vi "Misc.vi"() -> ()   [LabVIEW 2018]
uses:
  <vilib>/Rock Robotics/WPI/DriverStation/WPI_DriverStationRobotMode2.ctl
  <vilib>/Rock Robotics/Network Tables/NT Read Boolean.vi
  SubSystems/Drive Train/Drive Train Global.vi
  <vilib>/Rock Robotics/Network Tables/NT Read String.vi
  Robot Global Data.vi
  SubSystems/HAB Climber/HAB Climber Global.vi
  <vilib>/Rock Robotics/Network Tables/NT Write Boolean.vi
  SubSystems/Lift/Lift Global.vi
  SubSystems/Cargo Intake/Cargo Intake Global.vi
  SubSystems/Hatch Panel Intake/Hatch Panel Intake Global.vi
  <vilib>/Rock Robotics/Network Tables/NT Write Number.vi
  <vilib>/Rock Robotics/Network Tables/NT Write Numeric Array.vi
  Test Mode/Test Mode Global.vi
  <vilib>/Rock Robotics/Network Tables/NT Write Boolean Array.vi
  SubSystems/Controllers/Driver Controller/Driver Controller Global.vi
  SubSystems/Controllers/Manipulator Controlller/Manipulator Controller Global.vi
panel:
  in  "Boolean":bool=TRUE
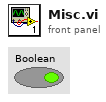
[diagram p1: front panel]
types:
  T1 = typedef "WPI_DriverStationRobotMode2.ctl" = enum16{"Autonomous Disabled", "Autonomous Enabled", "Teleop Disabled", "Teleop Enabled", "Disconnected", "Finish", "Test Disabled", "Test Enabled", "Emergency Stopped"}
  T2 = typedef "WPI_CompressorDevRef.ctl" = cluster{"DevStatus":errorcluster, "Pneumatics Control Module":u8}
  T3 = cluster{"FrontLeft":dbl, "FrontRight":dbl, "BackLeft":dbl, "BackRight":dbl}
  T4 = cluster{"Rollover":dbl, "Yaw":dbl, "Cont Yaw":dbl}
  T5 = cluster{"Drive Test?":bool, "Cargo Test?":bool, "Hatch Test?":bool, "Lift Test?":bool}
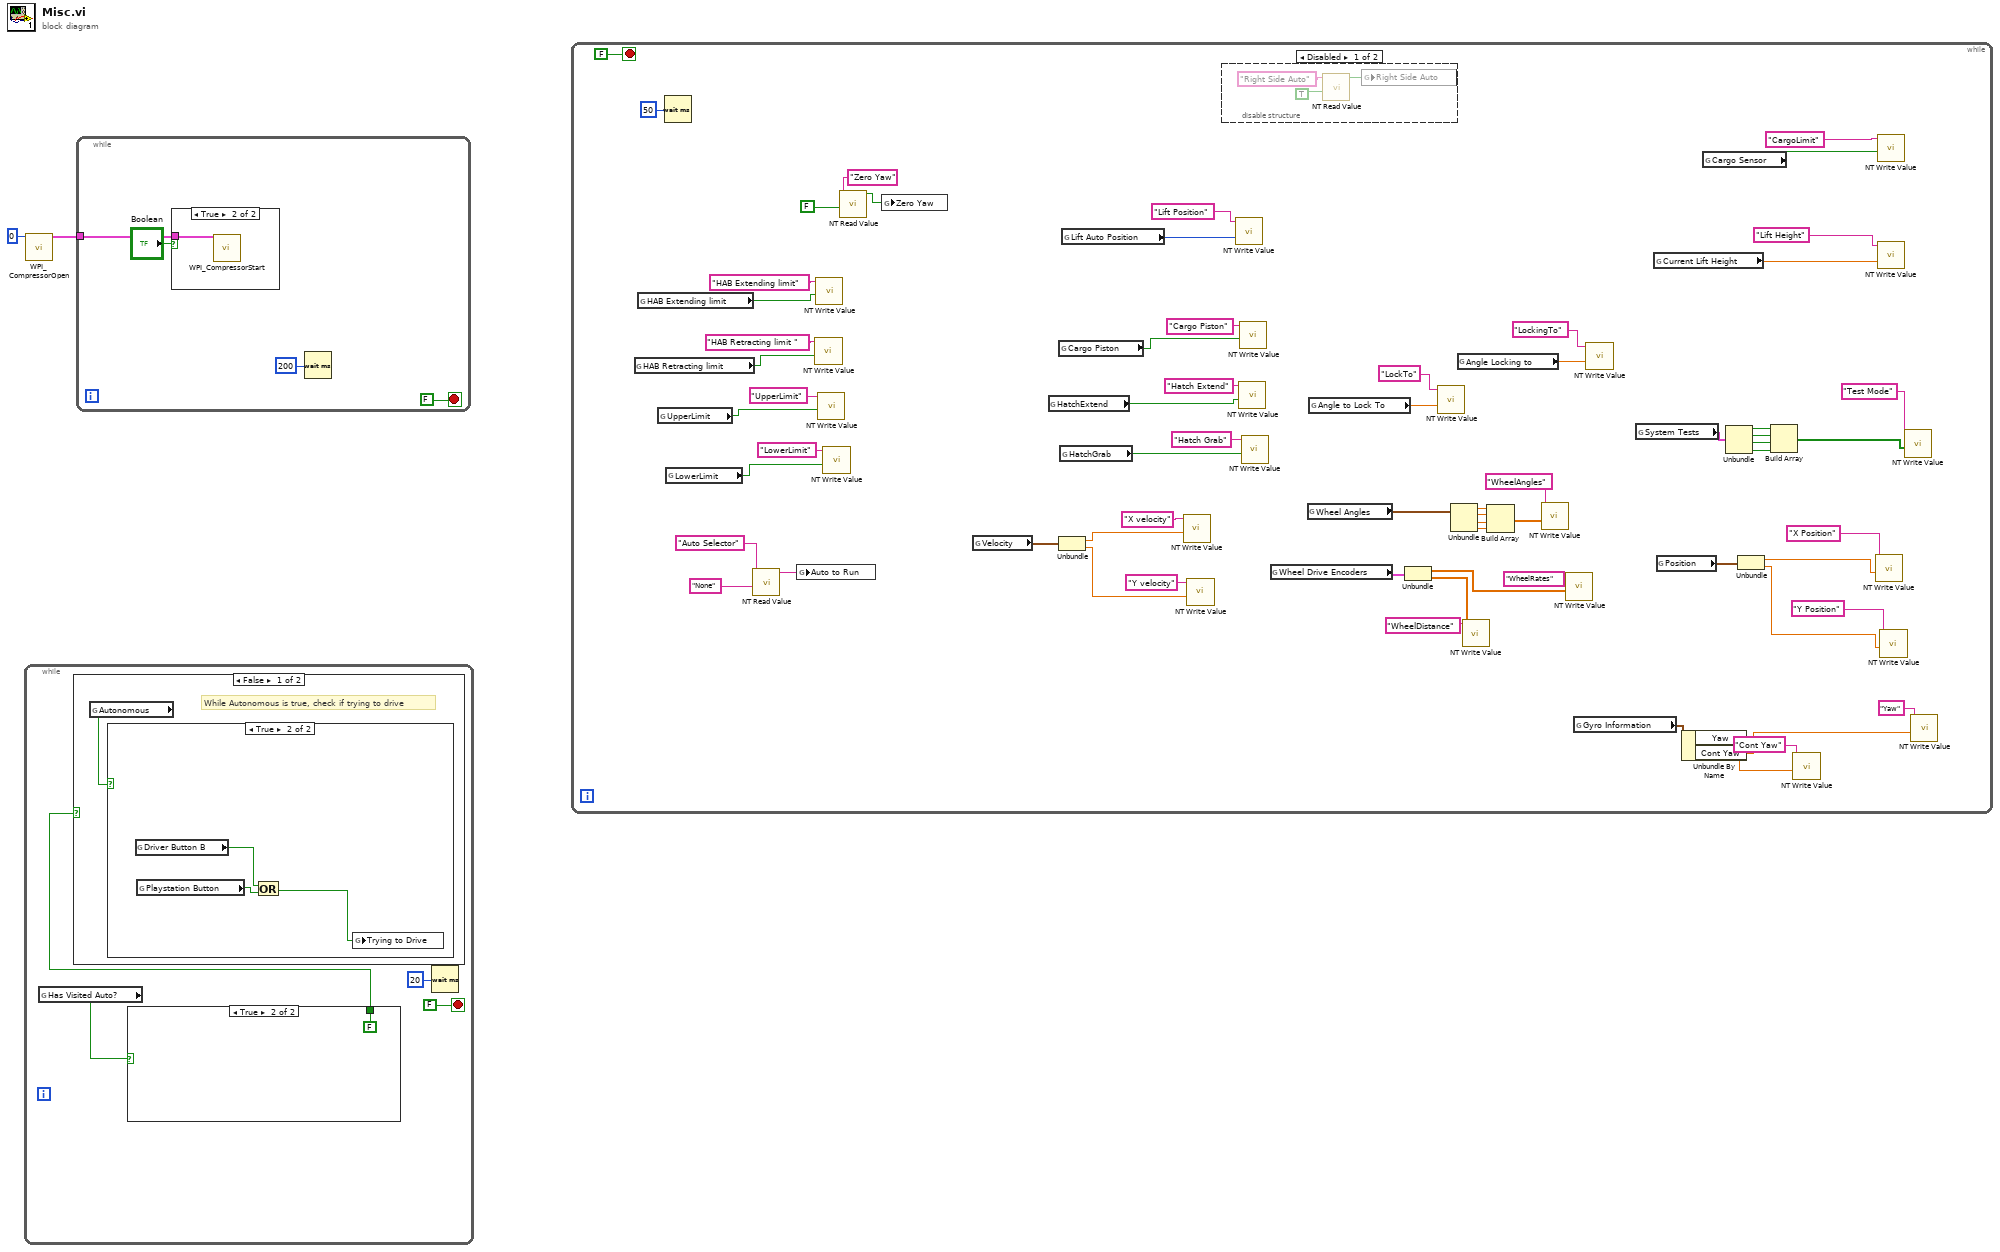
[diagram p0: block diagram]
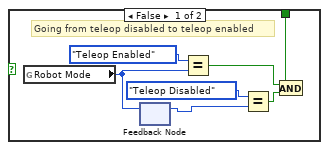
[diagram p2: hidden frame]
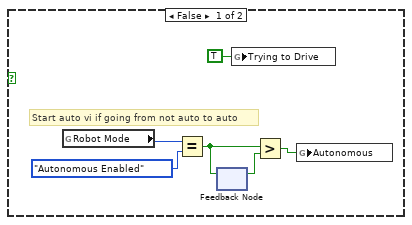
[diagram p3: hidden frame]
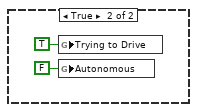
[diagram p4: hidden frame]
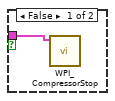
[diagram p6: hidden frame]
diagram:
  n1 = while {
    stop <- FALSE stop-if-true
    n2 = global read "Robot Global Data.vi" "Has Visited Auto?"() -> (w3:bool)
    n3 = case shown="True" w3 {
      tunnel: [w7 FALSE] -> w4
      frame False {
        # "Going from teleop disabled to teleop enabled"
        n4 = global read "Robot Global Data.vi" "Robot Mode"() -> (w13:T1)
        n5 = feedback #1() -> (w10:T1)  [unwired: 1 in]
        n6 = feedback-in #1(w13) -> ()
        n7 = Equal?(x=WPI_DriverStationRobotMode2."Teleop Enabled" ("y"), y=w13) -> (x = y?=w8:bool)
        n8 = Equal?(x=WPI_DriverStationRobotMode2."Teleop Disabled" ("y"), y=w10) -> (x = y?=w9:bool)
        n9 = And(x=w8, y=w9) -> (x .and. y?=w7:bool)
      }
      frame True {
      }
    }
    n10 = case shown="False" w4 {
      frame False {
        # "While Autonomous is true, check if trying to drive"
        n11 = global read "Robot Global Data.vi" "Autonomous"() -> (w15:bool)
        n12 = case shown="True" w15 {
          frame False {
            # "Start auto vi if going from not auto to auto"
            n13 = global read "Robot Global Data.vi" "Robot Mode"() -> (w17:T1)
            n14 = Equal?(x=w17, y=WPI_DriverStationRobotMode2."Autonomous Enabled") -> (x = y?=w18:bool)
            n15 = feedback #2() -> (w19:bool)  [unwired: 1 in]
            n16 = feedback-in #2(w18) -> ()
            n17 = global write "Robot Global Data.vi" "Trying to Drive"(TRUE ("Trying to Drive")) -> ()
            n18 = Greater?(x=w18, y=w19) -> (0:w20:bool)
            n19 = global write "Robot Global Data.vi" "Autonomous"(w20) -> ()
          }
          frame True {
            n20 = global read "Driver Controller Global.vi" "Driver Button B"() -> (w23:bool)
            n21 = global read "Manipulator Controller Global.vi" "Playstation Button"() -> (w22:bool)
            n22 = Compound Arithmetic op=OR(w23, w22) -> (w24:bool)
            n23 = global write "Robot Global Data.vi" "Trying to Drive"(w24) -> ()
          }
        }
      }
      frame True {
        n24 = global write "Robot Global Data.vi" "Trying to Drive"(TRUE ("Trying to Drive")) -> ()
        n25 = global write "Robot Global Data.vi" "Autonomous"(FALSE ("Autonomous")) -> ()
      }
    }
    n26 = Wait (ms)(milliseconds to wait=u32 20) -> ()  [unwired: 1 out]
  }
  n27 = call <vilib>:"WPI_CompressorOpen.vi"("Pneumatics Control Module (0)"=u8 0) -> ("CompressorDevRef"=w1:T2)  [unwired: 13 in, 1 out]
  n28 = while {
    tunnel: w1 -> [w29]
    stop <- FALSE stop-if-true
    n29 = case shown="True" "Boolean" {
      tunnel: w29 -> [w31 w32]
      frame False {
        n30 = call <vilib>:"WPI_CompressorStop.vi"("CompressorDevRef"=w31) -> ()  [unwired: 9 in, 2 out]
      }
      frame True {
        n31 = call <vilib>:"WPI_CompressorStart.vi"("CompressorDevRef"=w32) -> ()  [unwired: 9 in, 2 out]
      }
    }
    n32 = Wait (ms)(milliseconds to wait=u32 200) -> ()  [unwired: 1 out]
  }
  n33 = while {
    stop <- FALSE stop-if-true
    n34 = global read "HAB Climber Global.vi" "HAB Retracting limit"() -> (w89:bool)
    n35 = global read "HAB Climber Global.vi" "HAB Extending limit"() -> (w90:bool)
    n36 = global read "Lift Global.vi" "UpperLimit"() -> (w88:bool)
    n37 = Wait (ms)(milliseconds to wait=u32 50) -> ()  [unwired: 1 out]
    n38 = global read "Lift Global.vi" "LowerLimit"() -> (w87:bool)
    n39 = call-poly <vilib>:"NT Read Value.vi"("Default Value"="None", "Name"="Auto Selector") -> ("String"=w55:string)  [unwired: 8 in, 1 out]
    n40 = global write "Robot Global Data.vi" "Auto to Run"(w55) -> ()
    n41 = call-poly <vilib>:"NT Write Value.vi"("Boolean"=w89, "Name"="HAB Retracting limit ") -> ()  [unwired: 9 in, 1 out]
    n42 = call-poly <vilib>:"NT Write Value.vi"("Boolean"=w90, "Name"="HAB Extending limit") -> ()  [unwired: 9 in, 1 out]
    n43 = call-poly <vilib>:"NT Write Value.vi"("Boolean"=w88, "Name"="UpperLimit") -> ()  [unwired: 9 in, 1 out]
    n44 = call-poly <vilib>:"NT Write Value.vi"("Boolean"=w87, "Name"="LowerLimit") -> ()  [unwired: 9 in, 1 out]
    n45 = call-poly <vilib>:"NT Read Value.vi"("Default Value"=FALSE, "Name"="Zero Yaw") -> ("Boolean"=w95:bool)  [unwired: 8 in, 1 out]
    n46 = global write "Drive Train Global.vi" "Zero Yaw"(w95) -> ()
    n47 = global read "Drive Train Global.vi" "Velocity"() -> (w77:cluster{"X":dbl, "Y":dbl})
    n48 = global read "Hatch Panel Intake Global.vi" "HatchExtend"() -> (w81:bool)
    n49 = global read "Cargo Intake Global.vi" "Cargo Piston"() -> (w82:bool)
    n50 = Unbundle(w77) -> ("X"=w75:dbl, "Y"=w73:dbl)
    n51 = global read "Hatch Panel Intake Global.vi" "HatchGrab"() -> (w80:bool)
    n52 = global read "Lift Global.vi" "Lift Auto Position"() -> (w78:u16)
    n53 = call-poly <vilib>:"NT Write Value.vi"("Numeric"=w75, "Name"="X velocity") -> ()  [unwired: 9 in, 1 out]
    n54 = call-poly <vilib>:"NT Write Value.vi"("Numeric"=w73, "Name"="Y velocity") -> ()  [unwired: 9 in, 1 out]
    n55 = disable-structure shown="Disabled" {
      frame Disabled {
        n56 = call-poly <vilib>:"NT Read Value.vi"("Default Value"=TRUE, "Name"="Right Side Auto") -> ("Boolean"=w100:bool)  [unwired: 8 in, 1 out]
        n57 = global write "Robot Global Data.vi" "Right Side Auto"(w100) -> ()
      }
      frame Enabled {
      }
    }
    n58 = call-poly <vilib>:"NT Write Value.vi"("Numeric"=w78, "Name"="Lift Position") -> ()  [unwired: 9 in, 1 out]
    n59 = call-poly <vilib>:"NT Write Value.vi"("Boolean"=w81, "Name"="Hatch Extend") -> ()  [unwired: 9 in, 1 out]
    n60 = call-poly <vilib>:"NT Write Value.vi"("Boolean"=w82, "Name"="Cargo Piston") -> ()  [unwired: 9 in, 1 out]
    n61 = call-poly <vilib>:"NT Write Value.vi"("Boolean"=w80, "Name"="Hatch Grab") -> ()  [unwired: 9 in, 1 out]
    n62 = global read "Drive Train Global.vi" "Wheel Drive Encoders"() -> (w65:cluster{"Rates":dbl[], "Distances":dbl[]})
    n63 = global read "Drive Train Global.vi" "Wheel Angles"() -> (w72:T3)
    n64 = global read "Drive Train Global.vi" "Angle to Lock To"() -> (w60:dbl)
    n65 = Unbundle(w65) -> ("Rates"=w62:dbl[], "Distances"=w36:dbl[])
    n66 = call-poly <vilib>:"NT Write Value.vi"("Numeric"=w60, "Name"="LockTo") -> ()  [unwired: 9 in, 1 out]
    n67 = Unbundle(w72) -> ("FrontLeft"=w68:dbl, "FrontRight"=w69:dbl, "BackLeft"=w70:dbl, "BackRight"=w71:dbl)
    n68 = global read "Drive Train Global.vi" "Angle Locking to"() -> (w59:dbl)
    n69 = call-poly <vilib>:"NT Write Value.vi"("Numeric Array"=w36, "Name"="WheelDistance") -> ()  [unwired: 9 in, 1 out]
    n70 = Build Array(w68, w69, w70, w71) -> (w67:dbl[])
    n71 = call-poly <vilib>:"NT Write Value.vi"("Numeric Array"=w67, "Name"="WheelAngles") -> ()  [unwired: 9 in, 1 out]
    n72 = call-poly <vilib>:"NT Write Value.vi"("Numeric Array"=w62, "Name"="WheelRates") -> ()  [unwired: 9 in, 1 out]
    n73 = global read "Drive Train Global.vi" "Gyro Information"() -> (w42:T4)
    n74 = call-poly <vilib>:"NT Write Value.vi"("Numeric"=w59, "Name"="LockingTo") -> ()  [unwired: 9 in, 1 out]
    n75 = global read "Test Mode Global.vi" "System Tests"() -> (w50:T5)
    n76 = global read "Lift Global.vi" "Current Lift Height"() -> (w52:dbl)
    n77 = global read "Drive Train Global.vi" "Position"() -> (w39:cluster{"X":dbl, "Y":dbl})
    n78 = Unbundle By Name(w42) -> ("Yaw"=w38:dbl, "Cont Yaw"=w40:dbl)
    n79 = global read "Cargo Intake Global.vi" "Cargo Sensor"() -> (w54:bool)
    n80 = Unbundle(w50) -> ("Drive Test?"=w49:bool, "Cargo Test?"=w48:bool, "Hatch Test?"=w47:bool, "Lift Test?"=w46:bool)
    n81 = Unbundle(w39) -> ("X"=w35:dbl, "Y"=w33:dbl)
    n82 = Build Array(w49, w48, w47, w46) -> (w44:bool[])
    n83 = call-poly <vilib>:"NT Write Value.vi"("Numeric"=w38, "Name"="Cont Yaw") -> ()  [unwired: 9 in, 1 out]
    n84 = call-poly <vilib>:"NT Write Value.vi"("Numeric"=w35, "Name"="X Position") -> ()  [unwired: 9 in, 1 out]
    n85 = call-poly <vilib>:"NT Write Value.vi"("Boolean"=w54, "Name"="CargoLimit") -> ()  [unwired: 9 in, 1 out]
    n86 = call-poly <vilib>:"NT Write Value.vi"("Numeric"=w52, "Name"="Lift Height") -> ()  [unwired: 9 in, 1 out]
    n87 = call-poly <vilib>:"NT Write Value.vi"("Numeric"=w33, "Name"="Y Position") -> ()  [unwired: 9 in, 1 out]
    n88 = call-poly <vilib>:"NT Write Value.vi"("Boolean Array"=w44, "Name"="Test Mode") -> ()  [unwired: 9 in, 1 out]
    n89 = call-poly <vilib>:"NT Write Value.vi"("Numeric"=w40, "Name"="Yaw") -> ()  [unwired: 9 in, 1 out]
  }
